vi "Convert Shift Direction to Cmd.vi"(7 "cursor?":bool=TRUE, 11 "direction":enum16{"left", "right"}(ring)) -> (3 "LCD data/cmd":u8)   [LabVIEW 2017, in "HD44780 Common.lvlib"]
uses:
  HD44780 Common.lvlib
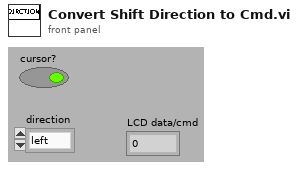
[diagram p1: front panel]
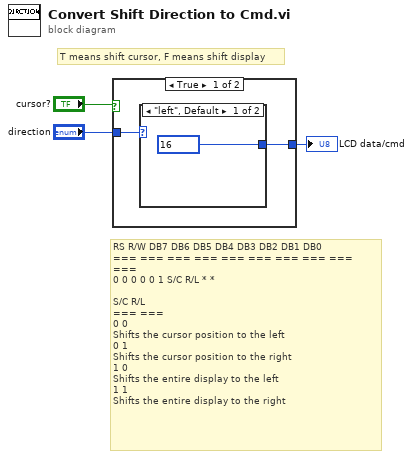
[diagram p0: block diagram]
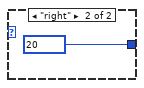
[diagram p2: hidden frame]
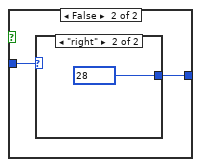
[diagram p3: hidden frame]
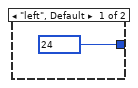
[diagram p4: hidden frame]
diagram:
  # "T means shift cursor, F means shift display"
  # "RS R/W DB7 DB6 DB5 DB4 DB3 DB2 DB1 DB0\n=== === === === === === === === === ===\n0 0 0 0 0 1 S/C R/L * *\n\nS/C R/L\n=== ===\n0 0 \nShifts the cursor position to the left\n0 1 \nShifts the cursor position to the right\n1 0 \nShifts the entire display to the left\n1 1 \nShifts the entire display to the right"
  n1 = case shown="True" "cursor?" {
    tunnel: [w5 w9] -> w3
    tunnel: "direction" -> [w4 w8]
    frame True {
      n2 = case shown="\"left\", Default" w4 {
        tunnel: [u8 16 ("LCD data/cmd") u8 20 ("LCD data/cmd")] -> w5
        frame "left", Default {
        }
        frame "right" {
        }
      }
    }
    frame False {
      n3 = case shown="\"right\"" w8 {
        tunnel: [u8 24 ("LCD data/cmd") u8 28 ("LCD data/cmd")] -> w9
        frame "left", Default {
        }
        frame "right" {
        }
      }
    }
  }
  "LCD data/cmd" <- w3
